vi "Get square wave duty cycle (%).vi"(8 "error in (no error)":errorcluster, 11 "Generator in":refnum<class "Generador.lvclass">) -> (0 "error out":errorcluster, 2 "square wave duty cycle (%)":dbl=50.0 format="%0.2f", 3 "Generator out":refnum<class "Generador.lvclass">)   [LabVIEW 2020, in "FGen.lvlib" / "Generador.lvclass"]
uses:
  Generador.lvclass
  Generador.lvclass/Generador.ctl
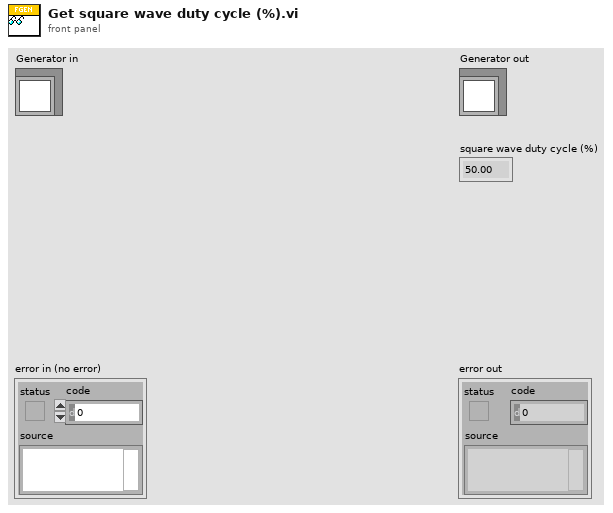
[diagram p1: front panel]
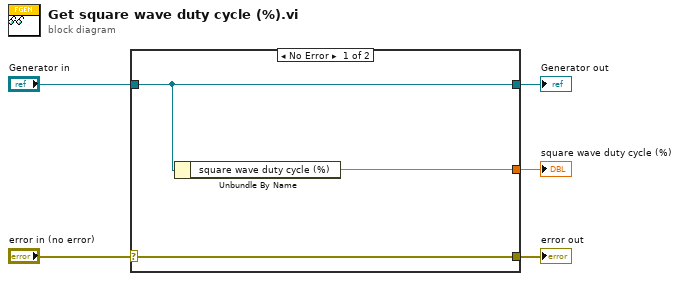
[diagram p0: block diagram]
diagram:
  n1 = case shown="No Error" "error in (no error)" {
    selector: "error in (no error)" -> [w8 w9]
    tunnel: [w8 w9] -> w4
    tunnel: [w7 w10] -> w2
    tunnel: "Generator in" -> [w7 w10]
    tunnel: [w6 _] -> w1
    frame No Error {
      n2 = Unbundle By Name(w7) -> ("square wave duty cycle (%)"=w6:dbl)
    }
    frame Error {
    }
  }
  "error out" <- w4
  "Generator out" <- w2
  "square wave duty cycle (%)" <- w1
